vi "Test App Error Handler is Configured for Immediate Parent of Nested Process.vi"(8 "error in (no error)":errorcluster, 11 "Rig Test In":refnum<class "Application Dev Test.lvclass">) -> (0 "error out":errorcluster, 3 "Rig Test Out":refnum<class "Application Dev Test.lvclass">)   [LabVIEW 2020, in "Application Dev Test.lvclass"]
uses:
  Application Dev Test.lvclass
  C:/Program Files (x86)/National Instruments/LabVIEW 2020/vi.lib/Astemes/LUnit/Test Case.lvclass
  source/Framework Test Suite/Mock Process/Mock Process.lvclass
  C:/Git/astemes-triarc-framework/source/Framework/Process/Process.lvclass
  source/Framework/Application/Application.lvclass
  source/Framework Test Suite/Mock Error Handler/Mock Error Handler.lvclass
  C:/Git/astemes-triarc-framework/source/Framework/Error Handler Interface/Error Handler Interface.lvclass
  source/Framework/Process/Process.lvclass/Process.ctl
  source/Framework/Application/Application.lvclass/Application.ctl
  <vilib>/Astemes/LUnit/Test Case.lvclass/Test Case.ctl
  <vilib>/Astemes/LUnit/LUnit Assertion Result.lvclass/LUnit Assertion Result.ctl
  <vilib>/Astemes/LUnit/LUnit Test Case Result.lvclass/LUnit Test Case Result.ctl
  <vilib>/Astemes/LUnit/LUnit Method Result.lvclass/LUnit Method Result.ctl
  a7f8edbc-9df4-4d07-9086-f8799b189c72.vi
  source/Framework/Application/Private/Add Process to Map.vi
  source/Framework/Application/Private/Start Idle Processes if Running.vi
  source/Framework/Application/Private/Throw Error If Process Already in App.vi
  source/Framework/Process/Protected/Messaging/Send Message.vi
  source/Framework/Process/Public/Lifecycle/Get Lifecycle State.vi
  source/Framework/Process/Protected/SubVIs/Set Context.vi
  source/Framework/Application/Private/Retrieve Process from App.vi
  source/Framework/Application/Private/Parse Process Name.vi
  source/Framework/Application/Private/Get Process from Map.vi
  <vilib>/Astemes/LUnit/Palette/Pass.vi
  <vilib>/Astemes/LUnit/Palette/Fail.vi
  <vilib>/Astemes/LUnit/Compare Variants.vi
  <vilib>/Astemes/LUnit/Describe Comparison.vi
  <vilib>/Astemes/LUnit/Set Assertion Type.vi
  source/Framework/Process/Private/SubVIs/Wait for finish.vi
  source/Framework/Process/Private/SubVIs/Set Lifecycle State.vi
  source/Framework/Process/Private/SubVIs/Handle Debug Data.vi
  <vilib>/Utility/error.llb/Clear Errors.vi
  source/Framework/Process/Public/Lifecycle/Leave Process Loop.vi
  source/Framework/Process/Protected/Messaging/Request Message.vi
  <vilib>/AdvancedString/Delimited String to 1D String Array.vi
  <vilib>/Astemes/LUnit/Add test result.vi
  <vilib>/Astemes/LUnit/LUnit Write Passed.vi
  <vilib>/Astemes/LUnit/LUnit Write Message.vi
  <vilib>/Astemes/LUnit/LUnit Write Description.vi
  <vilib>/Astemes/LUnit/Variant to string.vi
  <vilib>/Astemes/LUnit/LUnit Write Assertion Type.vi
  source/Framework/Logging/Log Debug.vi
  <vilib>/AdvancedString/1D String Array to Delimited String.vi
  <vilib>/Utility/High Resolution Relative Seconds.vi
  source/Framework/Process/Private/SubVIs/Enqueue Request Message.vi
  <vilib>/Astemes/LUnit/LUnit Record Assertion Result.vi
  <vilib>/Astemes/LUnit/LUnit Aggregate Assertion Results.vi
  <vilib>/Astemes/LUnit/Assertion Result/LUnit Read Status.vi
  <vilib>/Astemes/LUnit/LUnit Read Message.vi
  <vilib>/Astemes/LUnit/LUnit Read Description.vi
  <vilib>/Astemes/LUnit/Method Result/LUnit Merge Status.vi
  <vilib>/Astemes/LUnit/LUnit Concatenate result strings.vi
  <vilib>/Utility/error.llb/Error Cluster From Error Code.vi
  source/Framework/Process/Public/Read Name.vi
  source/Framework/Process/Private/SubVIs/Wait for Response Message.vi
  <vilib>/Utility/Data Type/Get Type Information.vi
  <vilib>/Utility/LVClass/Get LV Class Name.vi
  source/Framework/Process/Process.lvclass
  <vilib>/Astemes/LUnit/LUnit Assertion Result.lvclass
  Application Dev Test.lvclass/Application Dev Test.ctl
  <vilib>/Astemes/LUnit/Test Case.lvclass
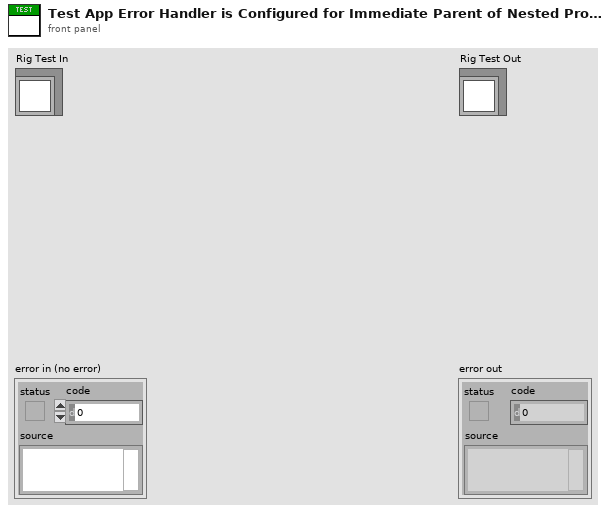
[diagram p1: front panel]
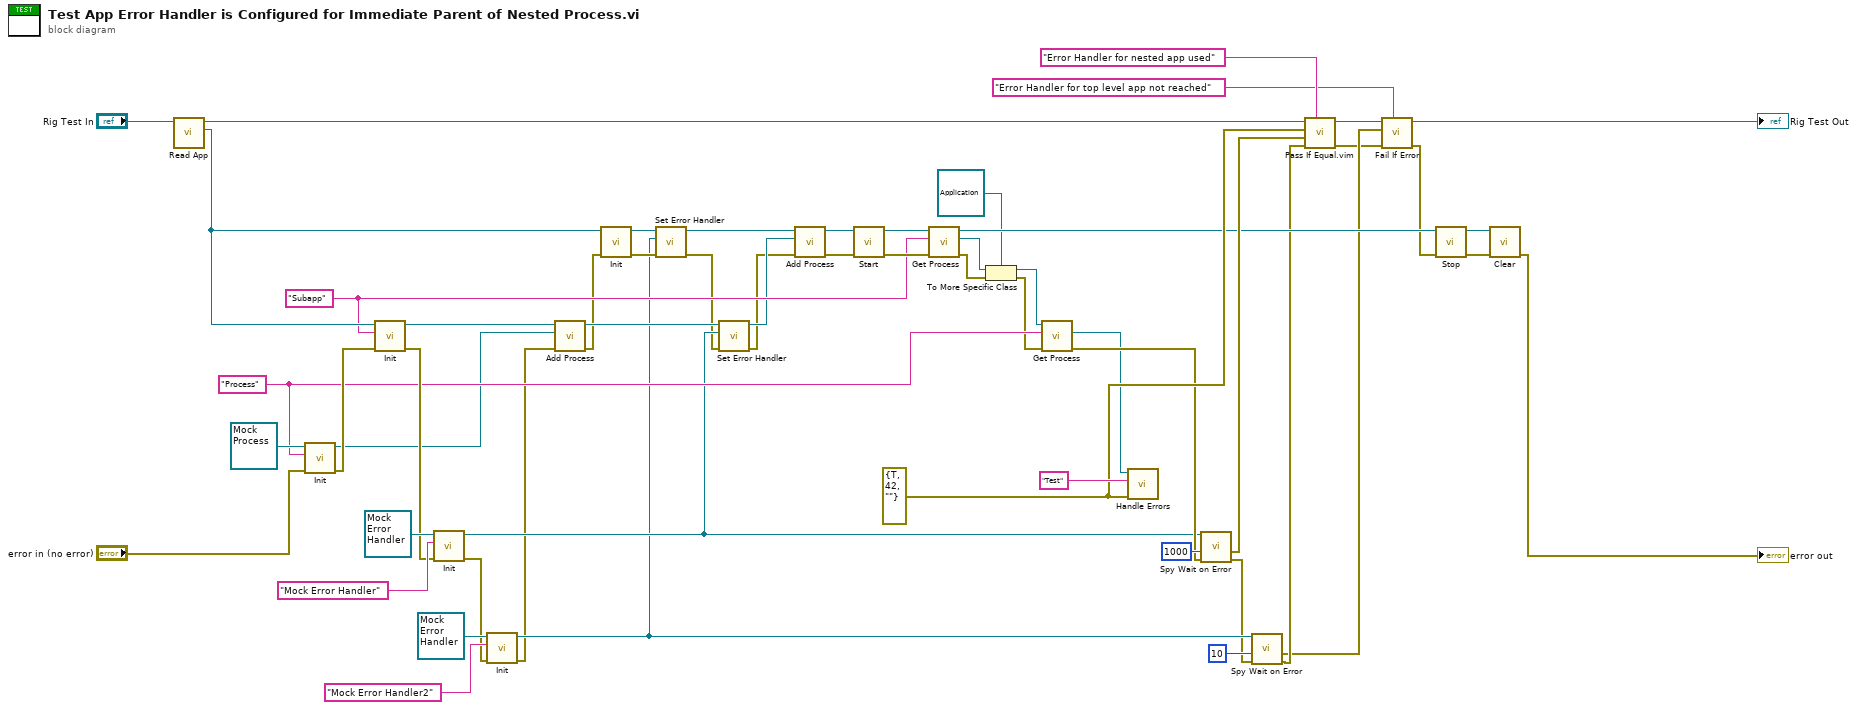
[diagram p0: block diagram]
diagram:
  w28 = "Subapp" ("Name")
  w45 = errorcluster {"status"=TRUE, "code"=42, "source"=""} ("error in (no error)")
  w41 = "Process" ("Name")
  n1 = call "Read App.vi"("Application Test In"="Rig Test In") -> ("App out"=w33:refnum<class "Application.lvclass">, "Application Test Out"=w52:refnum<class "Application Dev Test.lvclass">)  [unwired: 8 in, 1 out]
  n2 = call-dynamic "Init.vi"("error in (no error)"="error in (no error)", "Name"=w41, "Mock Process In"=refnum<class "Mock Process.lvclass"> refnum ("Mock Process.lvclass")) -> ("error out"=w49:errorcluster, "Mock Process Out"=w39:refnum<class "Mock Process.lvclass">)  [unwired: 7 in]
  n3 = call-dynamic "Init.vi"("error in (no error)"=w49, "Name"=w28, "Process In"=w33) -> ("error out"=w48:errorcluster, "Process Out"=w55:refnum<class "Application.lvclass">)  [unwired: 7 in]
  n4 = call-dynamic "Init.vi"("error in (no error)"=w48, "Name"="Mock Error Handler", "Mock Error Handler In"=refnum<class "Mock Error Handler.lvclass"> refnum ("Mock Error Handler.lvclass")) -> ("error out"=w10:errorcluster, "Mock Error Handler Out"=w18:refnum<class "Mock Error Handler.lvclass">)  [unwired: 7 in]
  n5 = call-dynamic "Init.vi"("error in (no error)"=w10, "Name"="Mock Error Handler2", "Mock Error Handler In"=refnum<class "Mock Error Handler.lvclass"> refnum ("Mock Error Handler.lvclass")) -> ("error out"=w9:errorcluster, "Mock Error Handler Out"=w11:refnum<class "Mock Error Handler.lvclass">)  [unwired: 7 in]
  n6 = call "Add Process.vi"("error in (no error)"=w9, "Process"=w39, "Application In"=w55) -> ("error out"=w17:errorcluster, "Application Out"=w20:refnum<class "Application.lvclass">)  [unwired: 7 in]
  n7 = call-dynamic "Init.vi"("error in (no error)"=w17, "Process In"=w33) -> ("error out"=w30:errorcluster, "Process Out"=w22:refnum<class "Application.lvclass">)  [unwired: 8 in]
  n8 = call "Set Error Handler.vi"("error in (no error)"=w30, "Error Handler"=w11, "Process In"=w22) -> ("error out"=w16:errorcluster, "Process Out"=w21:refnum<class "Application.lvclass">)  [unwired: 7 in]
  n9 = call "Set Error Handler.vi"("error in (no error)"=w16, "Error Handler"=w18, "Process In"=w20) -> ("error out"=w15:errorcluster, "Process Out"=w19:refnum<class "Application.lvclass">)  [unwired: 7 in]
  n10 = call "Add Process.vi"("error in (no error)"=w15, "Process"=w19, "Application In"=w21) -> ("error out"=w38:errorcluster, "Application Out"=w35:refnum<class "Application.lvclass">)  [unwired: 7 in]
  n11 = call "Start.vi"("error in (no error)"=w38, "Process In"=w35) -> ("error out"=w36:errorcluster, "Process Out"=w34:refnum<class "Application.lvclass">)  [unwired: 7 in, 1 out]
  n12 = call "Get Process.vi"("error in (no error)"=w36, "Process Name"=w28, "Application In"=w34) -> ("error out"=w25:errorcluster, "App Process"=w26:refnum<class "Process.lvclass">, "Application Out"=w29:refnum<class "Application.lvclass">)  [unwired: 6 in]
  n13 = To More Specific Class(target class=refnum<class "Application.lvclass"> refnum ("Rig Out"), reference=w26, error in=w25) -> (specific class reference=w23:refnum<class "Application.lvclass">, error out=w24:errorcluster)
  n14 = call "Get Process.vi"("error in (no error)"=w24, "Process Name"=w41, "Application In"=w23) -> ("error out"=w42:errorcluster, "App Process"=w40:refnum<class "Process.lvclass">)  [unwired: 6 in, 1 out]
  n15 = call-dynamic "Handle Errors.vi"("error in (no error)"=w45, "Location"="Test", "Process In"=w40) -> ()  [unwired: 7 in, 2 out]
  n16 = call "Spy Wait on Error.vi"("error in (no error)"=w42, "timeout in ms (-1)"=1000, "Mock Error Handler In"=w18) -> ("error out"=w5:errorcluster, "Errors"=w44:errorcluster)  [unwired: 4 in, 3 out]
  n17 = call "Spy Wait on Error.vi"("error in (no error)"=w5, "timeout in ms (-1)"=10, "Mock Error Handler In"=w11) -> ("error out"=w4:errorcluster, "Errors"=w3:errorcluster)  [unwired: 4 in, 3 out]
  n18 = call "Pass If Equal.vim"("Description"="Error Handler for nested app used", "error in (no error)"=w4, "Actual"=w44, "Expected"=w45, "LUnit Test Case In"=w52) -> ("error out"=w2:errorcluster, "LUnit Test Case Out"=w7:refnum<class "Application Dev Test.lvclass">)  [unwired: 5 in]
  n19 = call <vilib>:"Fail If Error.vi"("Description"="Error Handler for top level app not reached", "error in (no error)"=w2, "Assert error"=w3, "LUnit Test Case In"=w7) -> ("error out"=w8:errorcluster, "LUnit Test Case Out"=→"Rig Test Out":refnum<class "Application Dev Test.lvclass">)  [unwired: 6 in]
  n20 = call "Stop.vi"("error in (no error)"=w8, "Process In"=w29) -> ("error out"=w32:errorcluster, "Process Out"=w37:refnum<class "Application.lvclass">)  [unwired: 7 in, 1 out]
  n21 = call-dynamic "Clear.vi"("error in (no error)"=w32, "Application In"=w37) -> ("error out"=→"error out":errorcluster)  [unwired: 9 in]
